vi "SubVI_getSpectra_stable.vi"(1 "endPix":u16=3652, 2 "startPix":u16, 3 "test1":u8, 5 "Fast":u8, 7 "trigger":bool, 8 "keep trigger":bool, 9 "blank scans number":u8, 10 "scans number":u8=1, 11 "Exposure":u16=2) -> (0 "all spectra":u16[][](array[numeric]), 4 "Error":bool)   [LabVIEW 2022 SP3]
uses:
  adcDLL_0001.dll
panel:
  out "test count":i32
  in  "tot_startPix":u16=33
  in  "tot_endPix":u16=3685
  out "CountExposure":u16
  out "Count blanc":u8
  out "CountScans":u8
  out "program\nin process":bool
  out "Spectra 2":u16[](array[numeric])
  out "Spectra":u16[](array[numeric])
  out "InputReport1":u8[](array[numeric]) format="%x"
  out "Output Report":u8[](array[numeric])
  out "Input Report":u8[](array[numeric])
  # "test1 - \"1\" returne 0- 3711 (116*32)\n            \"0\" returne according to below\nFast -   \"0\" every pixel\n            \"1\" one out of 2 pixels in useful\n            information range"
  # "Move SRAM\ncount"
  # "384"
  # "useful information is in this range \n(already inside range of useful information)"
  # "useful information is in this range"
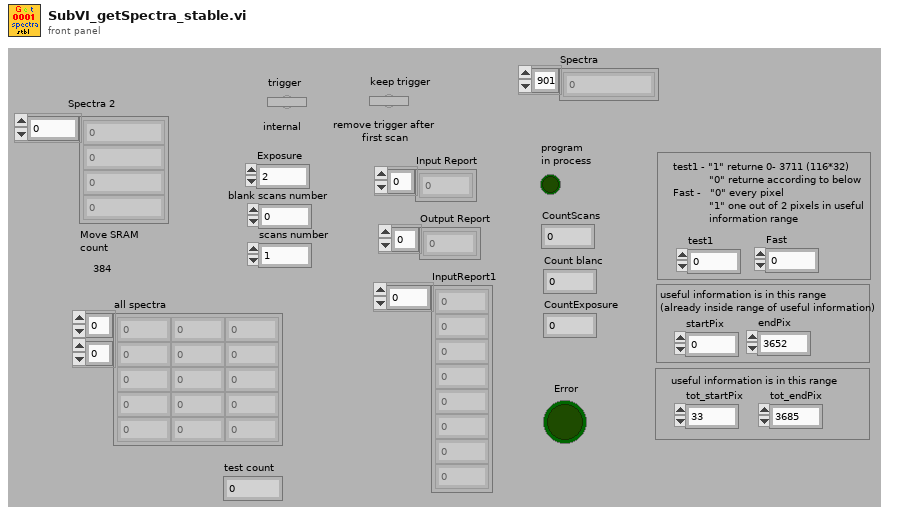
[diagram p1: front panel]
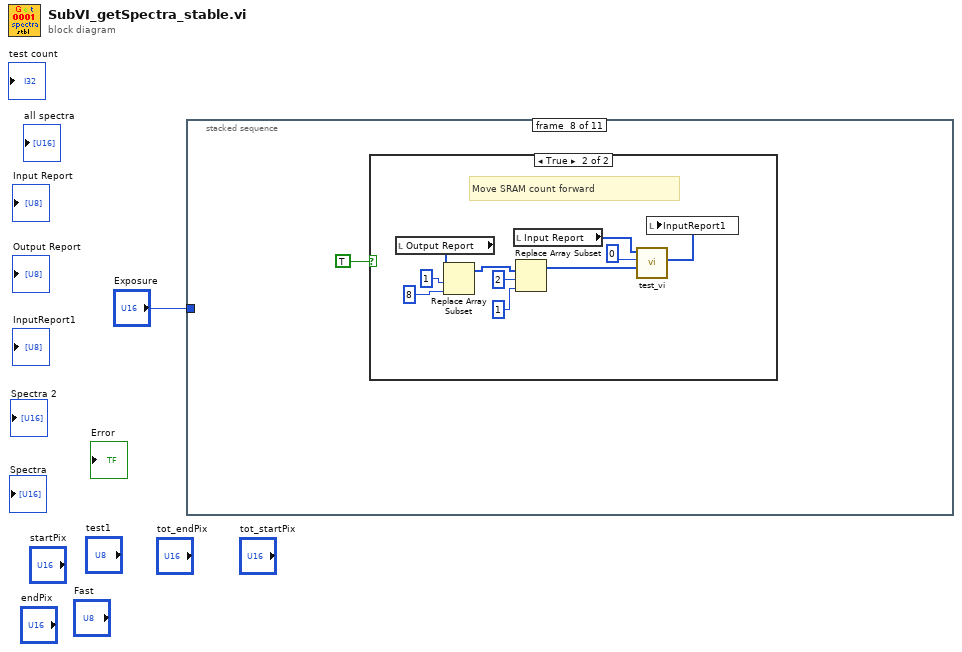
[diagram p0: block diagram]
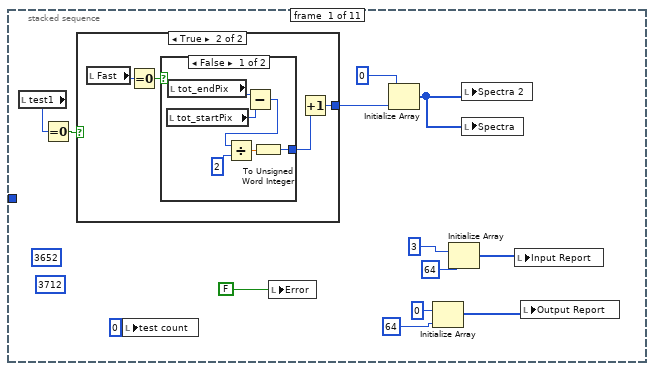
[diagram p2: hidden frame]
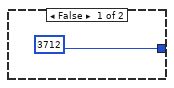
[diagram p3: hidden frame]
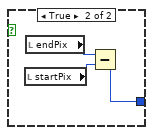
[diagram p4: hidden frame]
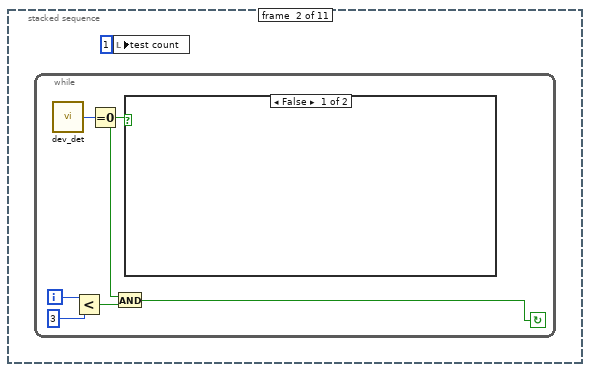
[diagram p5: hidden frame]
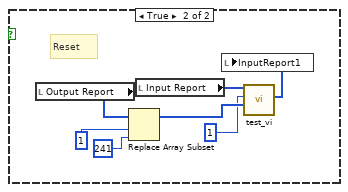
[diagram p6: hidden frame]
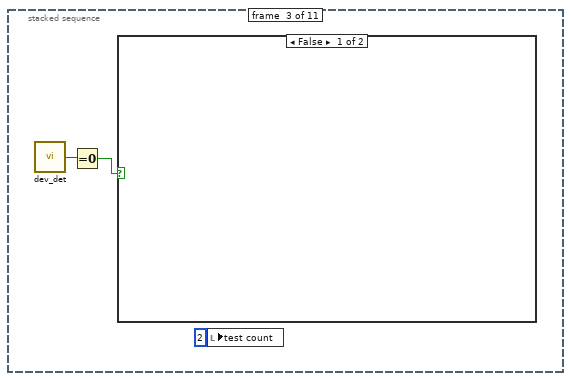
[diagram p7: hidden frame]
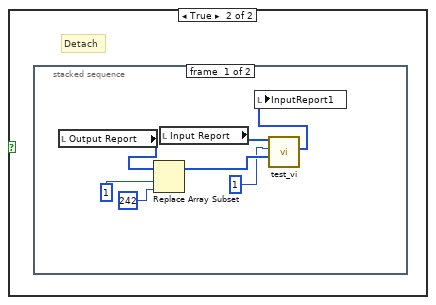
[diagram p8: hidden frame]
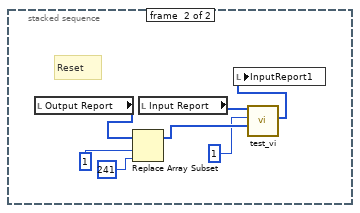
[diagram p9: hidden frame]
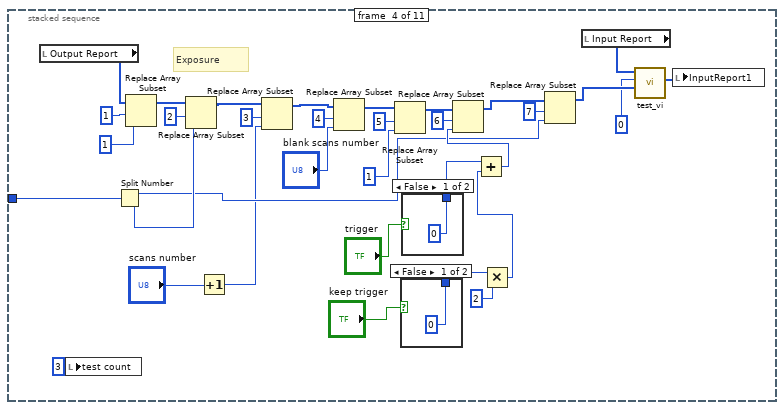
[diagram p10: hidden frame]
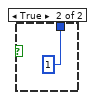
[diagram p11: hidden frame]
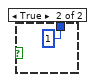
[diagram p12: hidden frame]
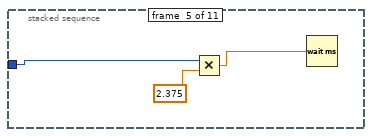
[diagram p13: hidden frame]
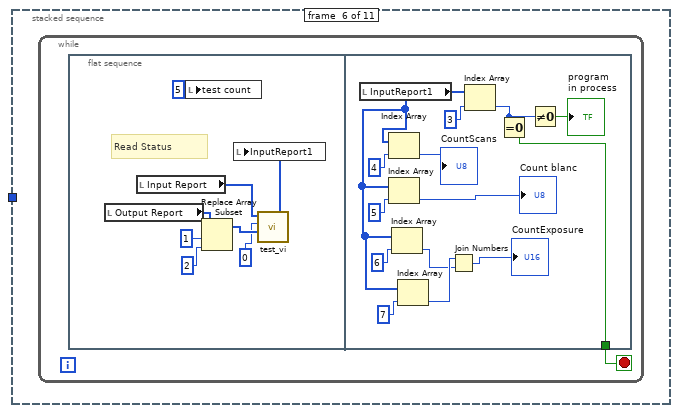
[diagram p14: hidden frame]
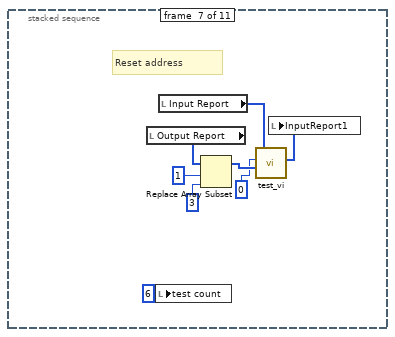
[diagram p15: hidden frame]
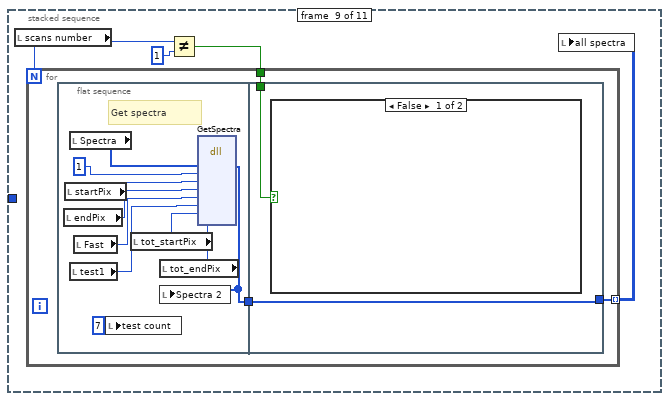
[diagram p17: hidden frame]
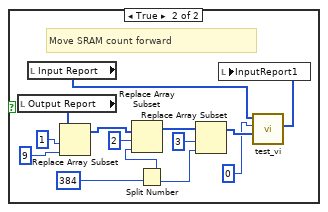
[diagram p18: hidden frame]
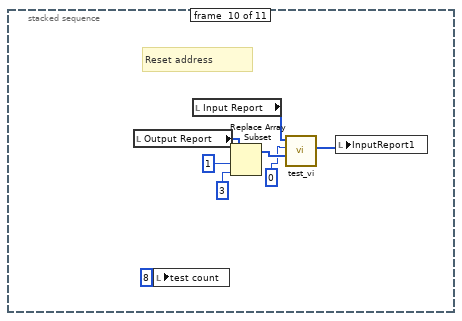
[diagram p19: hidden frame]
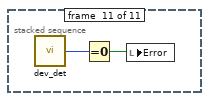
[diagram p20: hidden frame]
diagram:
  n1 = stacked-sequence {
    tunnel: "Exposure" -> [_ _ _ w65 w100 _ _ _ _ _ _]
    frame #0 {
      (unwired) u16 3712
      (unwired) 3652 ("dimension size")
      n2 = local read "test1"() -> (w6:u8)
      n3 = Equal To 0?(x=w6) -> (x = 0?=w5:bool)
      n4 = case shown="True" w5 {
        tunnel: [u16 3712 w16] -> w4
        frame False {
        }
        frame True {
          n5 = local read "Fast"() -> (w19:u8)
          n6 = Equal To 0?(x=w19) -> (x = 0?=w18:bool)
          n7 = case shown="False" w18 {
            tunnel: [w23 w28] -> w17
            frame False {
              n8 = local read "tot_startPix"() -> (w22:u16)
              n9 = local read "tot_endPix"() -> (w21:u16)
              n10 = Subtract(x=w21, y=w22) -> (x-y=w20:u16)
              n11 = Divide(x=w20, y=u16 2) -> (x/y=w24:dbl)
              n12 = To Unsigned Word Integer(number=w24) -> (unsigned 16bit integer=w23:u16)
            }
            frame True {
              n13 = local read "startPix"() -> (w26:u16)
              n14 = local read "endPix"() -> (w27:u16)
              n15 = Subtract(x=w27, y=w26) -> (x-y=w28:u16)
            }
          }
          n16 = Increment(x=w17) -> (x+1=w16:u16)
        }
      }
      n17 = local write "test count"(0 ("test count")) -> ()
      n18 = local write "Error"(FALSE ("Boolean")) -> ()
      n19 = Initialize Array(u16 0 ("element"), w4) -> (w13:u16[])
      n20 = Initialize Array(u8 0 ("element"), 64 ("dimension size")) -> (w7:u8[])
      n21 = Initialize Array(u8 3 ("element"), 64 ("dimension size")) -> (w8:u8[])
      n22 = local write "Spectra 2"(w13) -> ()
      n23 = local write "Spectra"(w13) -> ()
      n24 = local write "Input Report"(w8) -> ()
      n25 = local write "Output Report"(w7) -> ()
    }
    frame #1 {
      n26 = while {
        i -> [w34]
        stop <- w30 continue-if-true
        n27 = call "dev_det.vi"() -> ("DevDetect 2"=w35:u8)
        n28 = Less?(x=w34, y=3) -> (x < y?=w32:bool)
        n29 = Equal To 0?(x=w35) -> (x = 0?=w31:bool)
        n30 = And(x=w31, y=w32) -> (x .and. y?=w30:bool)
        n31 = case shown="False" w31 {
          frame False {
          }
          frame True {
            # "Reset"
            n32 = local read "Output Report"() -> (w40:u8[])
            n33 = Replace Array Subset(array=w40, new element=u8 241 ("new element/subarray"), index=1) -> (w41:u8[])
            n34 = local read "Input Report"() -> (w39:u8[])
            n35 = call "test_vi.vi"("OutputReport_in"=w41, "DevDet_in"=1, "InputReport_in"=w39) -> ("InputReport_out"=w42:u8[])  [unwired: 1 in, 3 out]
            n36 = local write "InputReport1"(w42) -> ()
          }
        }
      }
      n37 = local write "test count"(1 ("test count")) -> ()
    }
    frame #2 {
      n38 = call "dev_det.vi"() -> ("DevDetect 2"=w45:u8)
      n39 = Equal To 0?(x=w45) -> (x = 0?=w44:bool)
      n40 = case shown="False" w44 {
        frame False {
        }
        frame True {
          # "Detach"
          n41 = stacked-sequence {
            frame #0 {
              n42 = local read "Output Report"() -> (w50:u8[])
              n43 = Replace Array Subset(array=w50, new element=u8 242 ("new element/subarray"), index=1) -> (w47:u8[])
              n44 = local read "Input Report"() -> (w51:u8[])
              n45 = call "test_vi.vi"("OutputReport_in"=w47, "DevDet_in"=1, "InputReport_in"=w51) -> ("InputReport_out"=w52:u8[])  [unwired: 1 in, 3 out]
              n46 = local write "InputReport1"(w52) -> ()
            }
            frame #1 {
              # "Reset"
              n47 = local read "Output Report"() -> (w57:u8[])
              n48 = Replace Array Subset(array=w57, new element=u8 241 ("new element/subarray"), index=1) -> (w54:u8[])
              n49 = local read "Input Report"() -> (w58:u8[])
              n50 = call "test_vi.vi"("OutputReport_in"=w54, "DevDet_in"=1, "InputReport_in"=w58) -> ("InputReport_out"=w59:u8[])  [unwired: 1 in, 3 out]
              n51 = local write "InputReport1"(w59) -> ()
            }
          }
        }
      }
      n52 = local write "test count"(2 ("test count")) -> ()
    }
    frame #3 {
      # "Exposure"
      n53 = local read "Output Report"() -> (w91:u8[])
      n54 = local write "test count"(3 ("test count")) -> ()
      n55 = Split Number(x=w65) -> (hi(x)=w64:u8, lo(x)=w66:u8)
      n56 = Replace Array Subset(array=w91, new element=u8 1 ("new element/subarray"), index=1) -> (w93:u8[])
      n57 = Replace Array Subset(array=w93, new element=w66, index=2) -> (w85:u8[])
      n58 = Increment(x="scans number") -> (x+1=w60:u8)
      n59 = Replace Array Subset(array=w85, new element=w60, index=3) -> (w82:u8[])
      n60 = Replace Array Subset(array=w82, new element="blank scans number", index=4) -> (w80:u8[])
      n61 = Replace Array Subset(array=w80, new element=1 ("index"), index=5) -> (w77:u8[])
      n62 = case shown="False" "keep trigger" {
        tunnel: [0 ("index") 1 ("index")] -> w73
        frame False {
        }
        frame True {
        }
      }
      n63 = case shown="False" "trigger" {
        tunnel: [0 ("index") 1 ("index")] -> w71
        frame False {
        }
        frame True {
        }
      }
      n64 = Multiply(x=w73, y=2 ("index")) -> (x*y=w72:i32)
      n65 = Add(x=w71, y=w72) -> (x+y=w70:i32)
      n66 = Replace Array Subset(array=w77, new element=w70, index=6) -> (w67:u8[])
      n67 = Replace Array Subset(array=w67, new element=w64, index=7) -> (w63:u8[])
      n68 = local read "Input Report"() -> (w88:u8[])
      n69 = call "test_vi.vi"("OutputReport_in"=w63, "DevDet_in"=0, "InputReport_in"=w88) -> ("InputReport_out"=w87:u8[])  [unwired: 1 in, 3 out]
      n70 = local write "InputReport1"(w87) -> ()
    }
    frame #4 {
      n71 = Multiply(x=w100, y=2.375) -> (x*y=w98:dbl)
      n72 = Wait (ms)(milliseconds to wait=w98) -> ()  [unwired: 1 out]
    }
    frame #5 {
      n73 = while {
        stop <- w101 stop-if-true
        n74 = flat-sequence {
          tunnel: [w122] -> w101
          frame #0 {
            # "Read Status"
            n75 = local read "Output Report"() -> (w107:u8[])
            n76 = local read "Input Report"() -> (w108:u8[])
            n77 = local write "test count"(5 ("test count")) -> ()
            n78 = Replace Array Subset(array=w107, new element=u8 2 ("new element/subarray"), index=1) -> (w103:u8[])
            n79 = call "test_vi.vi"("OutputReport_in"=w103, "DevDet_in"=0, "InputReport_in"=w108) -> ("InputReport_out"=w109:u8[])  [unwired: 1 in, 3 out]
            n80 = local write "InputReport1"(w109) -> ()
          }
          frame #1 {
            n81 = local read "InputReport1"() -> (w113:u8[])
            n82 = Index Array(array=w113, index=4) -> (element=→"CountScans":u8)
            n83 = Index Array(array=w113, index=5) -> (element=→"Count blanc":u8)
            n84 = Index Array(array=w113, index=6) -> (element=w111:u8)
            n85 = Index Array(array=w113, index=7) -> (element=w112:u8)
            n86 = Join Numbers(hi=w112, lo=w111) -> ((hi.lo)=→"CountExposure":u16)
            n87 = Index Array(array=w113, index=3) -> (element=w121:u8)
            n88 = Equal To 0?(x=w121) -> (x = 0?=w122:bool)
            n89 = Not Equal To 0?(x=w121) -> (x != 0?=→"program\nin process":bool)
          }
        }
      }
    }
    frame #6 {
      # "Reset address"
      n90 = local read "Output Report"() -> (w129:u8[])
      n91 = local write "test count"(6 ("test count")) -> ()
      n92 = local read "Input Report"() -> (w130:u8[])
      n93 = Replace Array Subset(array=w129, new element=u8 3 ("new element/subarray"), index=1) -> (w125:u8[])
      n94 = call "test_vi.vi"("OutputReport_in"=w125, "DevDet_in"=0, "InputReport_in"=w130) -> ("InputReport_out"=w131:u8[])  [unwired: 1 in, 3 out]
      n95 = local write "InputReport1"(w131) -> ()
    }
    frame #7 {
      n96 = case shown="True" TRUE {
        frame False {
        }
        frame True {
          # "Move SRAM count forward"
          n97 = local read "Output Report"() -> (w140:u8[])
          n98 = Replace Array Subset(array=w140, new element=u8 8 ("new element/subarray"), index=1) -> (w138:u8[])
          n99 = local read "Input Report"() -> (w141:u8[])
          n100 = Replace Array Subset(array=w138, new element=u8 1, index=2) -> (w134:u8[])
          n101 = call "test_vi.vi"("OutputReport_in"=w134, "DevDet_in"=0, "InputReport_in"=w141) -> ("InputReport_out"=w142:u8[])  [unwired: 1 in, 3 out]
          n102 = local write "InputReport1"(w142) -> ()
        }
      }
    }
    frame #8 {
      n103 = local read "scans number"() -> (w144:u8)
      n104 = Not Equal?(x=w144, y=u8 1) -> (x != y?=w143:bool)
      n105 = for {
        N: w144 -> [_]
        tunnel: [w149] -> w146 mode=indexing
        tunnel: w143 -> [w147]
        n106 = flat-sequence {
          tunnel: [w159] -> w148
          tunnel: [w161] -> w149
          tunnel: w148 -> [w161]
          tunnel: w147 -> [w160]
          frame #0 {
            # "Get spectra"
            n107 = local read "endPix"() -> (w155:u16)
            n108 = local read "startPix"() -> (w156:u16)
            n109 = local read "Spectra"() -> (w158:u16[])
            n110 = local read "test1"() -> (w153:u8)
            n111 = local read "Fast"() -> (w154:u8)
            n112 = local write "test count"(7 ("test count")) -> ()
            n113 = local read "tot_startPix"() -> (w151:u16)
            n114 = local read "tot_endPix"() -> (w152:u16)
            n115 = dll-call lib="D:/LabVIEWSuite_64_OS/Spectrometers/ASEQ LR1/adcDLL_0001.dll" fn="GetSpectra"("InputSpec1"=w158, "SpecNmb"=u8 1, "startPix"=w156, "endPix"=w155, "Fast"=w154, "test1"=w153, "tot_startPix"=w151, "tot_endPix"=w152) -> ("InputSpec1"=w159:u16[])  [unwired: 11 in, 2 out]
            n116 = local write "Spectra 2"(w159) -> ()
          }
          frame #1 {
            n117 = case shown="False" w160 {
              frame False {
              }
              frame True {
                # "Move SRAM count forward"
                n118 = local read "Output Report"() -> (w175:u8[])
                n119 = local read "Input Report"() -> (w172:u8[])
                n120 = Replace Array Subset(array=w175, new element=u8 9 ("new element/subarray"), index=1) -> (w168:u8[])
                n121 = Split Number(x=u16 384) -> (hi(x)=w169:u8, lo(x)=w166:u8)
                n122 = Replace Array Subset(array=w168, new element=w169, index=2) -> (w165:u8[])
                n123 = Replace Array Subset(array=w165, new element=w166, index=3) -> (w163:u8[])
                n124 = call "test_vi.vi"("OutputReport_in"=w163, "DevDet_in"=0, "InputReport_in"=w172) -> ("InputReport_out"=w171:u8[])  [unwired: 1 in, 3 out]
                n125 = local write "InputReport1"(w171) -> ()
              }
            }
          }
        }
      }
      n126 = local write "all spectra"(w146) -> ()
    }
    frame #9 {
      # "Reset address"
      n127 = local read "Output Report"() -> (w182:u8[])
      n128 = local write "test count"(8 ("test count")) -> ()
      n129 = local read "Input Report"() -> (w181:u8[])
      n130 = Replace Array Subset(array=w182, new element=u8 3 ("new element/subarray"), index=1) -> (w177:u8[])
      n131 = call "test_vi.vi"("OutputReport_in"=w177, "DevDet_in"=0, "InputReport_in"=w181) -> ("InputReport_out"=w183:u8[])  [unwired: 1 in, 3 out]
      n132 = local write "InputReport1"(w183) -> ()
    }
    frame #10 {
      n133 = call "dev_det.vi"() -> ("DevDetect 2"=w185:u8)
      n134 = Equal To 0?(x=w185) -> (x = 0?=w184:bool)
      n135 = local write "Error"(w184) -> ()
    }
  }
